vi "SerialMonitor.vi"(8 "error in":errorcluster, 11 "VISA resource name in":refnum<visa-resource-name>) -> (0 "error out":errorcluster, 3 "VISA resource name out":refnum<visa-resource-name>)   [LabVIEW 2017]
panel:
  out "read buffer":string
  in  "Stop Button":bool
  in  "Enter":bool
  in  "Value":dbl
  in  "Value 1/2":enum16{"1", "2"}(ring)
  in  "Index":enum16{"1", "2", "3"}(ring)
  in  "Function":T1(ring)
  in  "SetGet":enum16{"Get", "Set"}(ring)
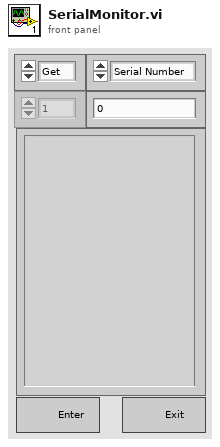
[diagram p1: front panel]
types:
  T1 = enum16{"Serial Number", "Temperature", "Unit Adress", "Calibration", "Velocity"}
  T2 = enum8{"Enabled", "Disabled", "Disabled and Grayed Out"}
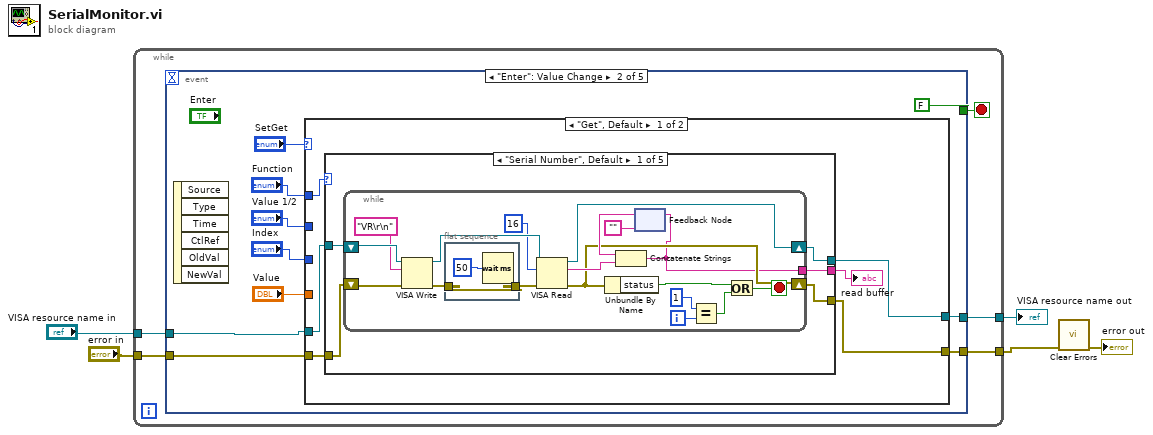
[diagram p0: block diagram]
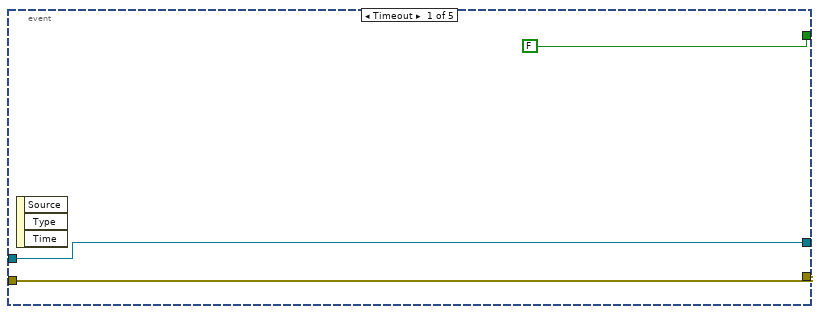
[diagram p2: hidden frame]
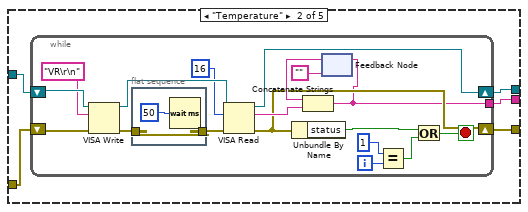
[diagram p3: hidden frame]
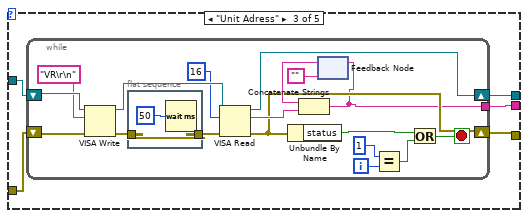
[diagram p4: hidden frame]
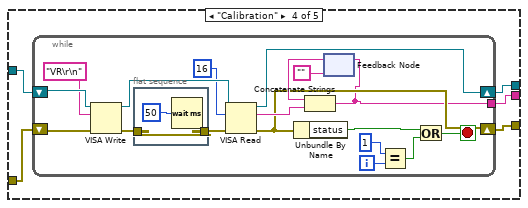
[diagram p5: hidden frame]
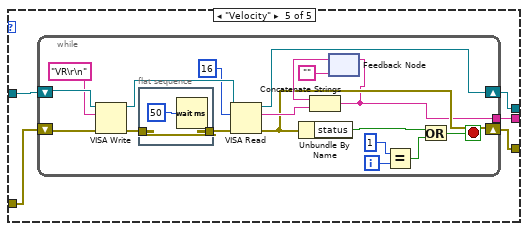
[diagram p6: hidden frame]
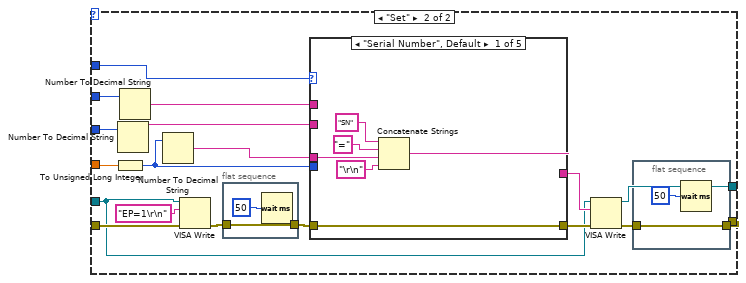
[diagram p7: hidden frame]
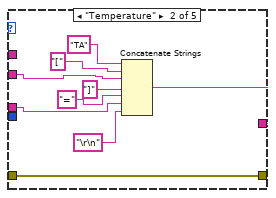
[diagram p8: hidden frame]
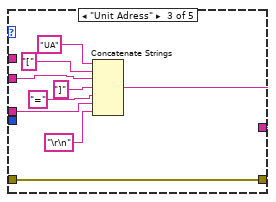
[diagram p9: hidden frame]
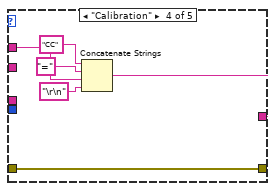
[diagram p10: hidden frame]
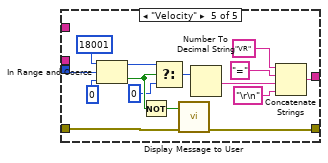
[diagram p11: hidden frame]
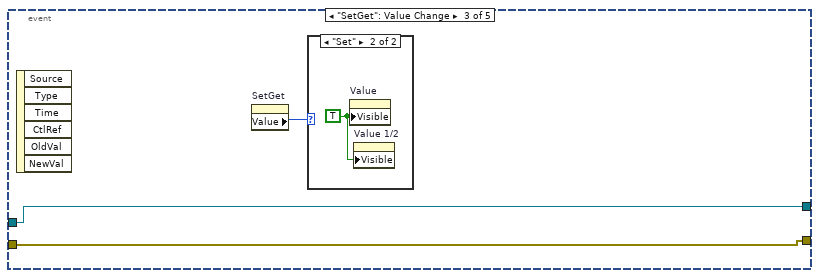
[diagram p12: hidden frame]
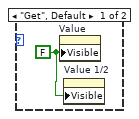
[diagram p13: hidden frame]
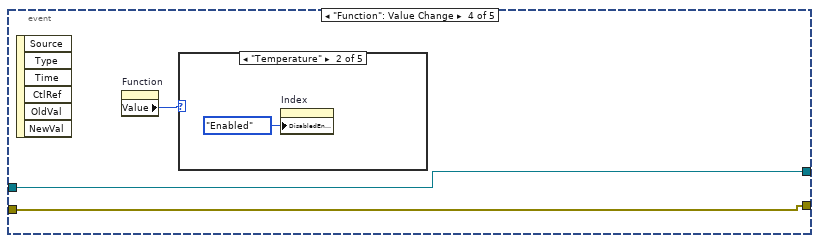
[diagram p14: hidden frame]
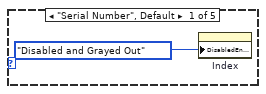
[diagram p15: hidden frame]
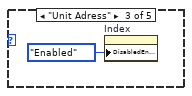
[diagram p16: hidden frame]
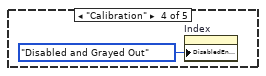
[diagram p17: hidden frame]
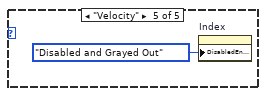
[diagram p18: hidden frame]
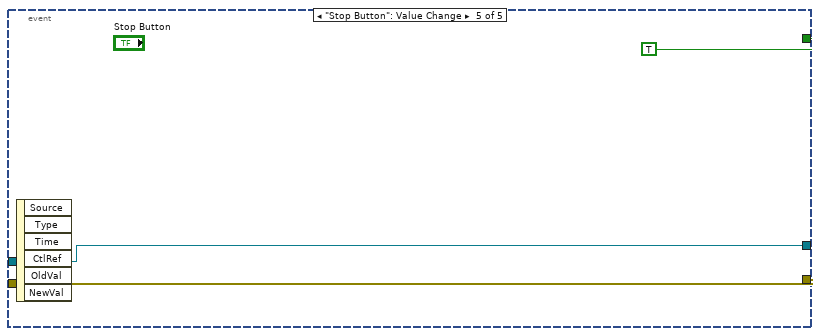
[diagram p19: hidden frame]
diagram:
  n1 = while {
    tunnel: "VISA resource name in" -> [w10]
    tunnel: "error in" -> [w9]
    tunnel: [w7] -> w1
    tunnel: [w6] -> w2
    stop <- w8 stop-if-true
    n2 = event shown="[1] \"Enter\": Value Change" {
      selector: _ -> [_ _ _ _ _]
      dyn-events: _ -> [_ _ _ _ _]
      timeout: _ -> [_ _ _ _ _]
      tunnel: w10 -> [w12 w20 w223 w228 w236]
      tunnel: w9 -> [w11 w19 w222 w227 w235]
      tunnel: [FALSE FALSE _ _ TRUE] -> w8
      tunnel: [w12 w15 w223 w228 w236] -> w7
      tunnel: [w11 w14 w222 w227 w235] -> w6
      event Timeout {
        n3 = event-data() -> ()  [unwired: 1 in, 3 out]
      }
      event "Enter": Value Change {
        n4 = event-data() -> ()  [unwired: 1 in, 6 out]
        n5 = case shown="\"Get\", Default" "SetGet" {
          tunnel: "Function" -> [w29 w172]
          tunnel: w20 -> [w28 w164]
          tunnel: w19 -> [w27 w169]
          tunnel: "Value" -> [_ w163]
          tunnel: "Value 1/2" -> [_ w161]
          tunnel: "Index" -> [_ w158]
          tunnel: [w26 w156] -> w15
          tunnel: [w25 w155] -> w14
          frame "Get", Default {
            n6 = case shown="\"Serial Number\", Default" w29 {
              tunnel: w28 -> [w34 w59 w84 w109 w134]
              tunnel: w27 -> [w33 w58 w83 w108 w133]
              tunnel: [w32 w57 w81 w107 w132] -> w26
              tunnel: [w31 w56 w82 w106 w131] -> w25
              tunnel: [w30 w55 w80 w105 w130] -> w24
              frame "Serial Number", Default {
                n7 = while {
                  shift-right: [w52] -> w32
                  shift-left: w34 -> [w51]
                  shift-right: [w39] -> w31
                  shift-left: w33 -> [w50]
                  tunnel: [w35] -> w30
                  i -> [w43]
                  stop <- w37 stop-if-true
                  n8 = VISA Write(VISA resource name=w51, write buffer="VR\r\n", error in (no error)=w50) -> (VISA resource name out=w49:refnum<visa-resource-name>, error out=w48:errorcluster)  [unwired: 1 out]
                  n9 = flat-sequence {
                    tunnel: w48 -> [w53]
                    tunnel: [w53] -> w47
                    frame #0 {
                      n10 = Wait (ms)(milliseconds to wait=u32 50) -> ()  [unwired: 1 out]
                    }
                  }
                  n11 = VISA Read(VISA resource name=w49, byte count=u32 16, error in (no error)=w47) -> (VISA resource name out=w52:refnum<visa-resource-name>, read buffer=w44:string, error out=w39:errorcluster)  [unwired: 1 out]
                  n12 = Unbundle By Name(w39) -> ("status"=w36:bool)
                  n13 = feedback #1("") -> (w46:string)
                  n14 = Concatenate Strings(w46, w44) -> (w35:string)
                  n15 = feedback-in #1(w35) -> ()
                  n16 = Equal?(x=1, y=w43) -> (x = y?=w38:bool)
                  n17 = Or(x=w36, y=w38) -> (x .or. y?=w37:bool)
                }
              }
              frame "Temperature" {
                n18 = while {
                  shift-right: [w77] -> w57
                  shift-left: w59 -> [w76]
                  shift-right: [w64] -> w56
                  shift-left: w58 -> [w75]
                  tunnel: [w60] -> w55
                  i -> [w68]
                  stop <- w62 stop-if-true
                  n19 = VISA Write(VISA resource name=w76, write buffer="VR\r\n", error in (no error)=w75) -> (VISA resource name out=w74:refnum<visa-resource-name>, error out=w73:errorcluster)  [unwired: 1 out]
                  n20 = flat-sequence {
                    tunnel: w73 -> [w78]
                    tunnel: [w78] -> w72
                    frame #0 {
                      n21 = Wait (ms)(milliseconds to wait=u32 50) -> ()  [unwired: 1 out]
                    }
                  }
                  n22 = VISA Read(VISA resource name=w74, byte count=u32 16, error in (no error)=w72) -> (VISA resource name out=w77:refnum<visa-resource-name>, read buffer=w69:string, error out=w64:errorcluster)  [unwired: 1 out]
                  n23 = Unbundle By Name(w64) -> ("status"=w61:bool)
                  n24 = feedback #2("") -> (w71:string)
                  n25 = Concatenate Strings(w71, w69) -> (w60:string)
                  n26 = feedback-in #2(w60) -> ()
                  n27 = Equal?(x=1, y=w68) -> (x = y?=w63:bool)
                  n28 = Or(x=w61, y=w63) -> (x .or. y?=w62:bool)
                }
              }
              frame "Unit Adress" {
                n29 = while {
                  shift-right: [w102] -> w81
                  shift-left: w84 -> [w101]
                  shift-right: [w89] -> w82
                  shift-left: w83 -> [w100]
                  tunnel: [w85] -> w80
                  i -> [w93]
                  stop <- w87 stop-if-true
                  n30 = VISA Write(VISA resource name=w101, write buffer="VR\r\n", error in (no error)=w100) -> (VISA resource name out=w99:refnum<visa-resource-name>, error out=w98:errorcluster)  [unwired: 1 out]
                  n31 = flat-sequence {
                    tunnel: w98 -> [w103]
                    tunnel: [w103] -> w97
                    frame #0 {
                      n32 = Wait (ms)(milliseconds to wait=u32 50) -> ()  [unwired: 1 out]
                    }
                  }
                  n33 = VISA Read(VISA resource name=w99, byte count=u32 16, error in (no error)=w97) -> (VISA resource name out=w102:refnum<visa-resource-name>, read buffer=w94:string, error out=w89:errorcluster)  [unwired: 1 out]
                  n34 = Unbundle By Name(w89) -> ("status"=w86:bool)
                  n35 = feedback #3("") -> (w96:string)
                  n36 = Concatenate Strings(w96, w94) -> (w85:string)
                  n37 = feedback-in #3(w85) -> ()
                  n38 = Equal?(x=1, y=w93) -> (x = y?=w88:bool)
                  n39 = Or(x=w86, y=w88) -> (x .or. y?=w87:bool)
                }
              }
              frame "Calibration" {
                n40 = while {
                  shift-right: [w127] -> w107
                  shift-left: w109 -> [w126]
                  shift-right: [w114] -> w106
                  shift-left: w108 -> [w125]
                  tunnel: [w110] -> w105
                  i -> [w118]
                  stop <- w112 stop-if-true
                  n41 = VISA Write(VISA resource name=w126, write buffer="VR\r\n", error in (no error)=w125) -> (VISA resource name out=w124:refnum<visa-resource-name>, error out=w123:errorcluster)  [unwired: 1 out]
                  n42 = flat-sequence {
                    tunnel: w123 -> [w128]
                    tunnel: [w128] -> w122
                    frame #0 {
                      n43 = Wait (ms)(milliseconds to wait=u32 50) -> ()  [unwired: 1 out]
                    }
                  }
                  n44 = VISA Read(VISA resource name=w124, byte count=u32 16, error in (no error)=w122) -> (VISA resource name out=w127:refnum<visa-resource-name>, read buffer=w119:string, error out=w114:errorcluster)  [unwired: 1 out]
                  n45 = Unbundle By Name(w114) -> ("status"=w111:bool)
                  n46 = feedback #4("") -> (w121:string)
                  n47 = Concatenate Strings(w121, w119) -> (w110:string)
                  n48 = feedback-in #4(w110) -> ()
                  n49 = Equal?(x=1, y=w118) -> (x = y?=w113:bool)
                  n50 = Or(x=w111, y=w113) -> (x .or. y?=w112:bool)
                }
              }
              frame "Velocity" {
                n51 = while {
                  shift-right: [w152] -> w132
                  shift-left: w134 -> [w151]
                  shift-right: [w139] -> w131
                  shift-left: w133 -> [w150]
                  tunnel: [w135] -> w130
                  i -> [w143]
                  stop <- w137 stop-if-true
                  n52 = VISA Write(VISA resource name=w151, write buffer="VR\r\n", error in (no error)=w150) -> (VISA resource name out=w149:refnum<visa-resource-name>, error out=w148:errorcluster)  [unwired: 1 out]
                  n53 = flat-sequence {
                    tunnel: w148 -> [w153]
                    tunnel: [w153] -> w147
                    frame #0 {
                      n54 = Wait (ms)(milliseconds to wait=u32 50) -> ()  [unwired: 1 out]
                    }
                  }
                  n55 = VISA Read(VISA resource name=w149, byte count=u32 16, error in (no error)=w147) -> (VISA resource name out=w152:refnum<visa-resource-name>, read buffer=w144:string, error out=w139:errorcluster)  [unwired: 1 out]
                  n56 = Unbundle By Name(w139) -> ("status"=w136:bool)
                  n57 = feedback #5("") -> (w146:string)
                  n58 = Concatenate Strings(w146, w144) -> (w135:string)
                  n59 = feedback-in #5(w135) -> ()
                  n60 = Equal?(x=1, y=w143) -> (x = y?=w138:bool)
                  n61 = Or(x=w136, y=w138) -> (x .or. y?=w137:bool)
                }
              }
            }
            "read buffer" <- w24
          }
          frame "Set" {
            n62 = To Unsigned Long Integer(number=w163) -> (unsigned 32bit integer=w159:u32)
            n63 = Number To Decimal String(number=w158) -> (decimal integer string=w157:string)  [unwired: 1 in]
            n64 = Number To Decimal String(number=w161) -> (decimal integer string=w160:string)  [unwired: 1 in]
            n65 = Number To Decimal String(number=w159) -> (decimal integer string=w162:string)  [unwired: 1 in]
            n66 = VISA Write(VISA resource name=w164, write buffer="EP=1\r\n", error in (no error)=w169) -> (error out=w170:errorcluster)  [unwired: 2 out]
            n67 = flat-sequence {
              tunnel: w170 -> [w175]
              tunnel: [w175] -> w166
              frame #0 {
                n68 = Wait (ms)(milliseconds to wait=u32 50) -> ()  [unwired: 1 out]
              }
            }
            n69 = case shown="\"Serial Number\", Default" w172 {
              tunnel: [w178 w184 w193 w201 w219] -> w168
              tunnel: w166 -> [w177 w183 w192 w206 w210]
              tunnel: [w177 w183 w192 w206 w207] -> w165
              tunnel: w162 -> [w179 w185 w198 _ _]
              tunnel: w160 -> [_ _ _ w202 _]
              tunnel: w159 -> [_ _ _ _ w211]
              tunnel: w157 -> [_ w186 w196 _ _]
              frame "Serial Number", Default {
                n70 = Concatenate Strings("SN" ("write buffer"), "=" ("string"), w179, "\r\n" ("write buffer")) -> (w178:string)
              }
              frame "Temperature" {
                n71 = Concatenate Strings("TA" ("string"), "[", w186, "]", "=" ("string"), w185, "\r\n" ("write buffer")) -> (w184:string)
              }
              frame "Unit Adress" {
                n72 = Concatenate Strings("UA" ("string"), "[", w196, "]", "=" ("string"), w198, "\r\n" ("write buffer")) -> (w193:string)
              }
              frame "Calibration" {
                n73 = Concatenate Strings("CC" ("string"), "=" ("string"), w202, "\r\n" ("write buffer")) -> (w201:string)
              }
              frame "Velocity" {
                n74 = In Range and Coerce(upper limit=u16 18001, x=w211, lower limit=u16 0) -> (coerced(x)=w217:u32, In Range?=w215:bool)
                n75 = Not(x=w215) -> (.not. x?=w216:bool)
                n76 = Select(t=w217, s=w215, f=u16 0) -> (s? t:f=w209:u32)
                n77 = call "Display Message to User"("error in (no error)"=w210, "Enable"=w216) -> ("error out"=w207:errorcluster)  [unwired: 8 in, 1 out]
                n78 = Number To Decimal String(number=w209) -> (decimal integer string=w208:string)  [unwired: 1 in]
                n79 = Concatenate Strings("VR" ("write buffer"), "=" ("string"), w208, "\r\n" ("write buffer")) -> (w219:string)
              }
            }
            n80 = VISA Write(VISA resource name=w164, write buffer=w168, error in (no error)=w165) -> (VISA resource name out=w156:refnum<visa-resource-name>, error out=w167:errorcluster)  [unwired: 1 out]
            n81 = flat-sequence {
              tunnel: w167 -> [w173]
              tunnel: [w173] -> w155
              frame #0 {
                n82 = Wait (ms)(milliseconds to wait=u32 50) -> ()  [unwired: 1 out]
              }
            }
          }
        }
      }
      event "SetGet": Value Change {
        n83 = event-data() -> ()  [unwired: 1 in, 6 out]
        n84 = property on="SetGet" class="Enum (strict)"() -> ("Value"=w224:enum16{"Get", "Set"})  [unwired: 2 in, 2 out]
        n85 = case shown="\"Set\"" w224 {
          frame "Get", Default {
            w225 = FALSE ("Visible")
            n86 = property on="Value" class="DigNum (strict)"("Visible"=w225) -> ()  [unwired: 2 in, 2 out]
            n87 = property on="Value 1/2" class="Enum (strict)"("Visible"=w225) -> ()  [unwired: 2 in, 2 out]
          }
          frame "Set" {
            w226 = TRUE ("Visible")
            n88 = property on="Value" class="DigNum (strict)"("Visible"=w226) -> ()  [unwired: 2 in, 2 out]
            n89 = property on="Value 1/2" class="Enum (strict)"("Visible"=w226) -> ()  [unwired: 2 in, 2 out]
          }
        }
      }
      event "Function": Value Change {
        n90 = event-data() -> ()  [unwired: 1 in, 6 out]
        n91 = property on="Function" class="Enum (strict)"() -> ("Value"=w229:T1)  [unwired: 2 in, 2 out]
        n92 = case shown="\"Temperature\"" w229 {
          frame "Serial Number", Default {
            n93 = property on="Index" class="Enum (strict)"("DisabledEnum"=T2."Disabled and Grayed Out" ("Disabled")) -> ()  [unwired: 2 in, 2 out]
          }
          frame "Temperature" {
            n94 = property on="Index" class="Enum (strict)"("DisabledEnum"=T2."Enabled" ("Disabled")) -> ()  [unwired: 2 in, 2 out]
          }
          frame "Unit Adress" {
            n95 = property on="Index" class="Enum (strict)"("DisabledEnum"=T2."Enabled" ("Disabled")) -> ()  [unwired: 2 in, 2 out]
          }
          frame "Calibration" {
            n96 = property on="Index" class="Enum (strict)"("DisabledEnum"=T2."Disabled and Grayed Out" ("Disabled")) -> ()  [unwired: 2 in, 2 out]
          }
          frame "Velocity" {
            n97 = property on="Index" class="Enum (strict)"("DisabledEnum"=T2."Disabled and Grayed Out" ("Disabled")) -> ()  [unwired: 2 in, 2 out]
          }
        }
      }
      event "Stop Button": Value Change {
        n98 = event-data() -> ()  [unwired: 1 in, 6 out]
      }
    }
  }
  "VISA resource name out" <- w1
  n99 = call <vilib>:"Clear Errors.vi"("error in (no error)"=w2) -> ("error out"=→"error out":errorcluster)  [unwired: 5 in, 1 out]
